vi "Check Bundler.vi"(8 "error in (no error)":errorcluster, 10 "Bundler":refnum<vi>, 11 "Search in":refnum<class "Search.lvclass">) -> (0 "error out":errorcluster, 2 "Match?":bool, 3 "Search out":refnum<class "Search.lvclass">)   [LabVIEW 2016, in "Better Search.lvlib" / "Search.lvclass"]
uses:
  Search.lvclass
  Better Search.lvlib
  <vilib>/regexp/Match Regular Expression.xnode
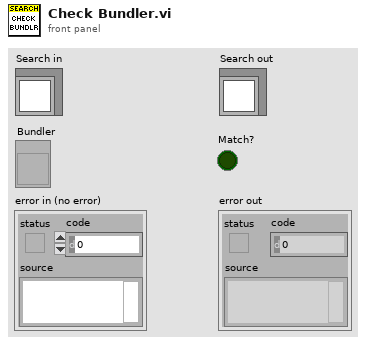
[diagram p1: front panel]
types:
  T1 = typedef "Better Search.lvlib/Search Type.ctl" = enum16{"Generic", "Text", "Data Type", "VI", "Node"}
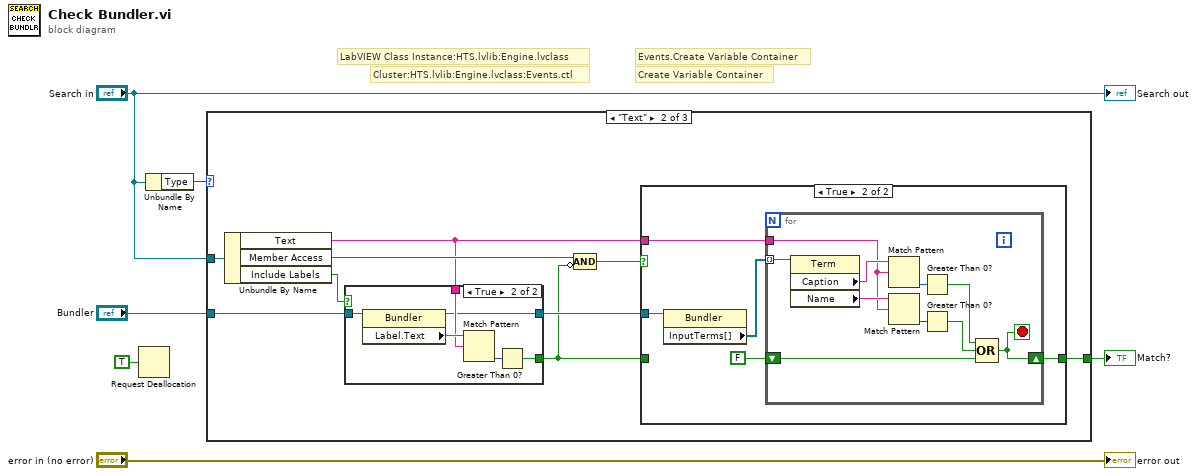
[diagram p0: block diagram]
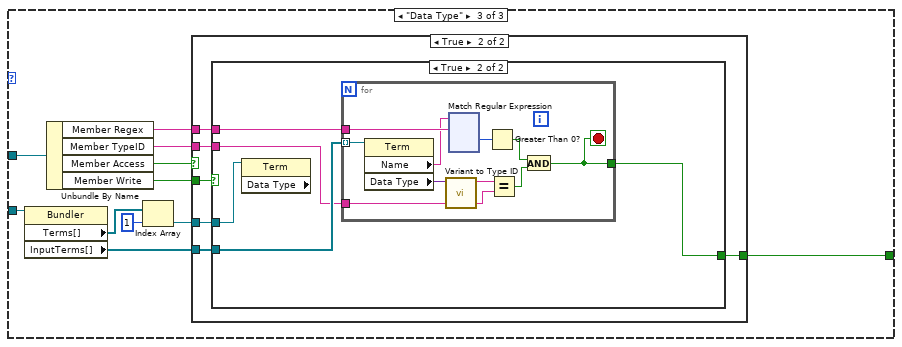
[diagram p5: hidden frame]
diagram:
  # "Cluster:HTS.lvlib:Engine.lvclass:Events.ctl"
  # "Create Variable Container"
  # "LabVIEW Class Instance:HTS.lvlib:Engine.lvclass"
  # "Events.Create Variable Container"
  n1 = Request Deallocation(TRUE ("flag")) -> ()
  n2 = Unbundle By Name("Search in") -> ("Type"=w5:T1)
  n3 = case shown="\"Text\"" w5 {
    tunnel: "Search in" -> [_ w15 w49]
    tunnel: [_ w13 w39] -> w3
    tunnel: "Bundler" -> [_ w10 w46]
    frame Default {
    }
    frame "Text" {
      n4 = Unbundle By Name(w15) -> ("Text"=w12:string, "Member Access"=w14:bool, "Include Labels"=w9:bool)
      n5 = case shown="True" w9 {
        tunnel: w12 -> [_ w20]
        tunnel: [w16 w19] -> w11
        tunnel: w10 -> [w16 w18]
        tunnel: [_ w17] -> w7
        frame False {
        }
        frame True {
          n6 = property class="Bundler"(reference=w18) -> (reference out=w19:refnum<vi>, "Label.Text"=w21:string)  [unwired: 1 in, 1 out]
          n7 = Match Pattern(string=w21, regular expression=w20) -> (offset past match=w22:i32)  [unwired: 1 in, 3 out]
          n8 = Greater Than 0?(x=w22) -> (x > 0?=w17:bool)
        }
      }
      n9 = Compound Arithmetic op=AND(w14, invert w7) -> (w8:bool)
      n10 = case shown="True" w8 {
        tunnel: w12 -> [_ w28]
        tunnel: [w23 w26] -> w13
        tunnel: w11 -> [_ w24]
        tunnel: w7 -> [w23 _]
        frame False {
        }
        frame True {
          n11 = property class="Bundler"(reference=w24) -> ("InputTerms[]"=w25:refnum<vi>[])  [unwired: 1 in, 2 out]
          n12 = for {
            tunnel: w25 -> [w38] mode=indexing
            tunnel: w28 -> [w35]
            shift-right: [w29] -> w26
            shift-left: FALSE -> [w34]
            stop <- w29 stop-if-true
            n13 = property class="Term"(reference=w38) -> ("Caption"=w37:string, "Name"=w36:string)  [unwired: 1 in, 2 out]
            n14 = Match Pattern(string=w37, regular expression=w35) -> (offset past match=w32:i32)  [unwired: 1 in, 3 out]
            n15 = Match Pattern(string=w36, regular expression=w35) -> (offset past match=w33:i32)  [unwired: 1 in, 3 out]
            n16 = Greater Than 0?(x=w32) -> (x > 0?=w31:bool)
            n17 = Greater Than 0?(x=w33) -> (x > 0?=w30:bool)
            n18 = Compound Arithmetic op=OR(w31, w30, w34) -> (w29:bool)
          }
        }
      }
    }
    frame "Data Type" {
      n19 = property class="Bundler"(reference=w46) -> ("Terms[]"=w45:refnum<vi>[], "InputTerms[]"=w42:refnum<vi>[])  [unwired: 1 in, 2 out]
      n20 = Unbundle By Name(w49) -> ("Member Regex"=w47:string, "Member TypeID"=w41:string, "Member Access"=w40:bool, "Member Write"=w48:bool)
      n21 = Index Array(array=w45, index=1) -> (element=w43:refnum<vi>)
      n22 = case shown="True" w40 {
        tunnel: w48 -> [_ w52]
        tunnel: w47 -> [_ w54]
        tunnel: w43 -> [_ w55]
        tunnel: w42 -> [_ w53]
        tunnel: w41 -> [_ w51]
        tunnel: [_ w50] -> w39
        frame False {
        }
        frame True {
          n23 = case shown="True" w52 {
            tunnel: w55 -> [_ w60]
            tunnel: w54 -> [_ w57]
            tunnel: w53 -> [_ w59]
            tunnel: w51 -> [_ w56]
            tunnel: [_ w58] -> w50
            frame False {
            }
            frame True {
              n24 = property class="Term" props=["Data Type"](reference=w60) -> ()  [unwired: 1 in, 3 out]
              n25 = for {
                tunnel: w59 -> [w70] mode=indexing
                tunnel: w57 -> [w64]
                tunnel: [w65] -> w58
                tunnel: w56 -> [w67]
                stop <- w65 stop-if-true
                n26 = property class="Term"(reference=w70) -> ("Name"=w63:string, "Data Type"=w69:variant)  [unwired: 1 in, 2 out]
                n27 = call "Variant to Type ID.vi"("Variant"=w69) -> ("Type ID"=w68:string)  [unwired: 9 in, 1 out]
                n28 = xnode "Match Regular Expression"("input string"=w63, "regular expression"=w64) -> ("offset past match"=w62:i32)  [unwired: 4 in, 4 out]
                n29 = Greater Than 0?(x=w62) -> (x > 0?=w61:bool)
                n30 = Equal?(x=w68, y=w67) -> (x = y?=w66:bool)
                n31 = And(x=w61, y=w66) -> (x .and. y?=w65:bool)
              }
            }
          }
        }
      }
    }
  }
  "Match?" <- w3
  "error out" <- "error in (no error)"
  "Search out" <- "Search in"
